vi "Show or Hide Front Panel.vi"(8 "error in (no error)":errorcluster, 10 "Show Front Panel?":bool, 11 "Person in":refnum<class "Person.lvclass">) -> (0 "error out":errorcluster, 3 "Person out":refnum<class "Person.lvclass">)   [LabVIEW 2023, in "Person.lvlib" / "Person.lvclass"]
doc: "Toggles whether the Front Panel is shown."
uses:
  Person.lvclass
  Person.lvclass/Person.ctl
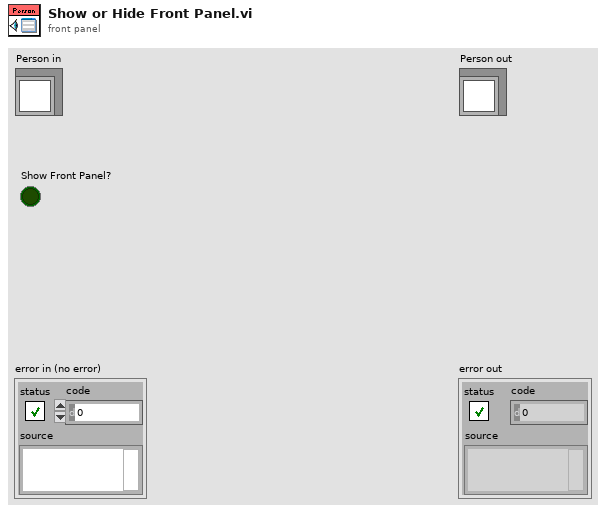
[diagram p1: front panel]
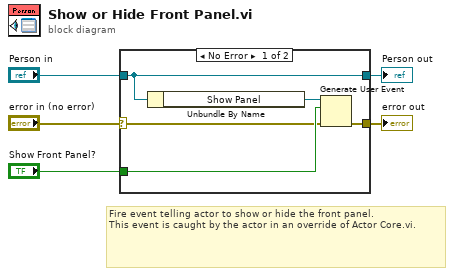
[diagram p0: block diagram]
diagram:
  # "Fire event telling actor to show or hide the front panel.\nThis event is caught by the actor in an override of Actor Core.vi."
  n1 = case shown="No Error" "error in (no error)" {
    selector: "error in (no error)" -> [w7 w12]
    tunnel: [w6 w12] -> w4
    tunnel: [w10 w11] -> w2
    tunnel: "Person in" -> [w10 w11]
    tunnel: "Show Front Panel?" -> [w8 _]
    frame No Error {
      n2 = Unbundle By Name(w10) -> ("Show Panel"=w9:refnum<user-event>)
      n3 = Generate User Event(user event=w9, event data cluster=w8, error in=w7) -> (error out=w6:errorcluster)  [unwired: 1 in, 1 out]
    }
    frame Error {
    }
  }
  "error out" <- w4
  "Person out" <- w2
